vi "Determine Warnings.vi"() -> ()   [LabVIEW 2014]
panel:
  out "Warning?":bool
  out "Warning Text":string
  in  "Min Temp 2":dbl
  in  "Max Temp":dbl
  in  "Current Temp":dbl
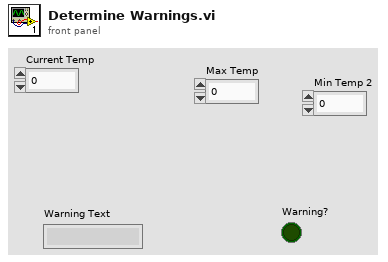
[diagram p1: front panel]
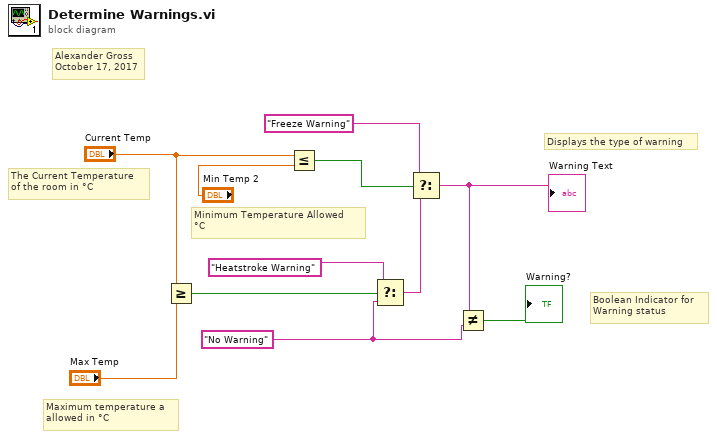
[diagram p0: block diagram]
diagram:
  w3 = "No Warning"
  # "Alexander Gross\nOctober 17, 2017"
  # "Displays the type of warning"
  # "Boolean Indicator for \nWarning status"
  # "Minimum Temperature Allowed\n°C"
  # "Maximum temperature a\nallowed in °C"
  # "The Current Temperature \nof the room in °C"
  n1 = Greater Or Equal?(x="Current Temp", y="Max Temp") -> (x >= y?=w8:bool)
  n2 = Less Or Equal?(x="Current Temp", y="Min Temp 2") -> (x <= y?=w6:bool)
  n3 = Select(t="Heatstroke Warning", s=w8, f=w3) -> (s? t:f=w4:string)
  n4 = Select(t="Freeze Warning", s=w6, f=w4) -> (s? t:f=w2:string)
  "Warning Text" <- w2
  n5 = Not Equal?(x=w2, y=w3) -> (x != y?=→"Warning?":bool)
